vi "circularCounter_v2.vi"(7 "reset":bool, 9 "doStep":bool=TRUE, 11 "maxCount":u16) -> (0 "maxReached":bool, 1 "maxPulse":bool, 2 "next":u16, 3 "index":u16)   [LabVIEW 2016]
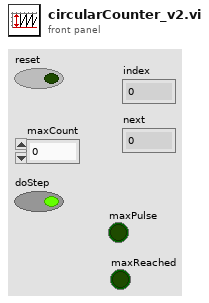
[diagram p1: front panel]
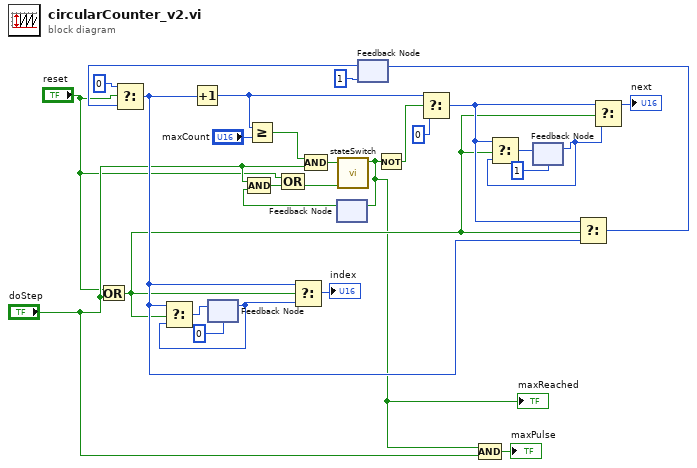
[diagram p0: block diagram]
diagram:
  n1 = Or(x="reset", y="doStep") -> (x .or. y?=w13:bool)
  n2 = feedback #1(u16 0 ("t")) -> (w20:u16)
  n3 = feedback #2() -> (w6:bool)  [unwired: 1 in]
  n4 = Compound Arithmetic op=AND("doStep", w6) -> (w7:bool)
  n5 = Compound Arithmetic op=OR("reset", w7) -> (w2:bool)
  n6 = feedback #3(u16 1) -> (w27:u16)
  n7 = Select(t=u16 0, s="reset", f=w27) -> (s? t:f=w21:u16)
  n8 = Select(t=w21, s=w13, f=w20) -> (s? t:f=w22:u16)
  n9 = Increment(x=w21) -> (x+1=w10:u16)
  n10 = feedback-in #1(w22) -> ()
  n11 = Greater Or Equal?(x=w10, y="maxCount") -> (x >= y?=w9:bool)
  n12 = Select(t=w21, s=w13, f=w20) -> (s? t:f=→"index":u16)
  n13 = Compound Arithmetic op=AND(w9, "doStep") -> (w8:bool)
  n14 = call "stateSwitch.vi"("disable"=w2, "enable"=w8) -> ("state"=w3:bool)  [unwired: 9 in]
  "maxReached" <- w3
  n15 = feedback-in #2(w3) -> ()
  n16 = Not(x=w3) -> (.not. x?=w4:bool)
  n17 = Select(t=w10, s=w4, f=u16 0) -> (s? t:f=w19:u16)
  n18 = Compound Arithmetic op=AND(w3, "doStep") -> (→"maxPulse":bool)
  n19 = feedback #4(u16 1) -> (w17:u16)
  n20 = Select(t=w19, s=w13, f=w17) -> (s? t:f=w18:u16)
  n21 = feedback-in #4(w18) -> ()
  n22 = Select(t=w19, s=w13, f=w21) -> (s? t:f=w25:u16)
  n23 = feedback-in #3(w25) -> ()
  n24 = Select(t=w19, s=w13, f=w17) -> (s? t:f=→"next":u16)
